vi "test_UDP Protocol Factory.vi"(8 "error in (no error)":errorcluster, 11 "TestCase in":refnum<class "Instrument Addon Scripting API Protocol Factories Unit Tests.lvclass">) -> (0 "error out":errorcluster, 3 "TestCase out":refnum<class "Instrument Addon Scripting API Protocol Factories Unit Tests.lvclass">)   [LabVIEW 2018, in "Instrument Addon Scripting API Protocol Factories Unit Tests.lvclass"]
uses:
  Instrument Addon Scripting API Protocol Factories Unit Tests.lvclass
  UDP/UDP Settings.ctl
  UDP/UDP.lvclass/UDP.ctl
  UDP/Data Access/Read Local IP Address.vi
  UDP/Data Access/Read Local Port.vi
  UDP/Data Access/Read Target IP Address.vi
  UDP/Data Access/Read Target Port.vi
  <vilib>/addons/_JKI Toolkits/VI Tester/TestCase.llb/TestCase.lvclass
  UDP/UDP.lvclass
  C:/Program Files (x86)/National Instruments/LabVIEW 2018/vi.lib/addons/_JKI Toolkits/VI Tester/TestCase.llb/TestCase.lvclass
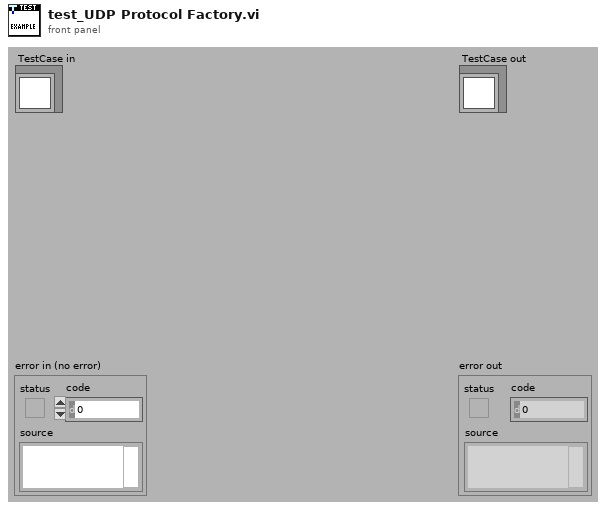
[diagram p1: front panel]
types:
  T1 = typedef "Protocols.lvlib/UDP.lvclass/UDP Settings.ctl" = cluster{"Local IP Address":string, "Local Port":u16, "Target IP Address":string, "Target Port":u16}
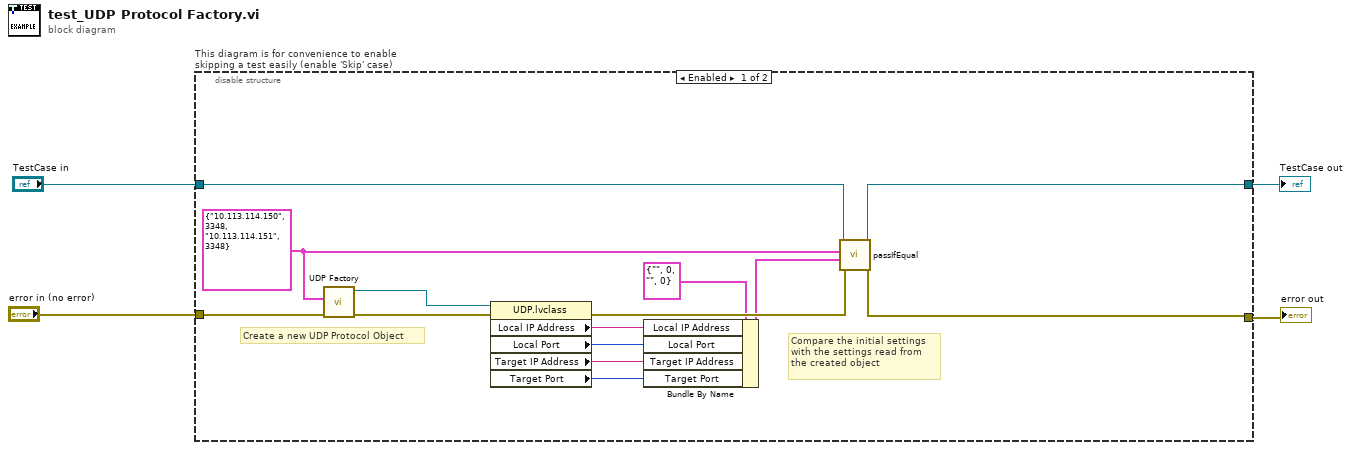
[diagram p0: block diagram]
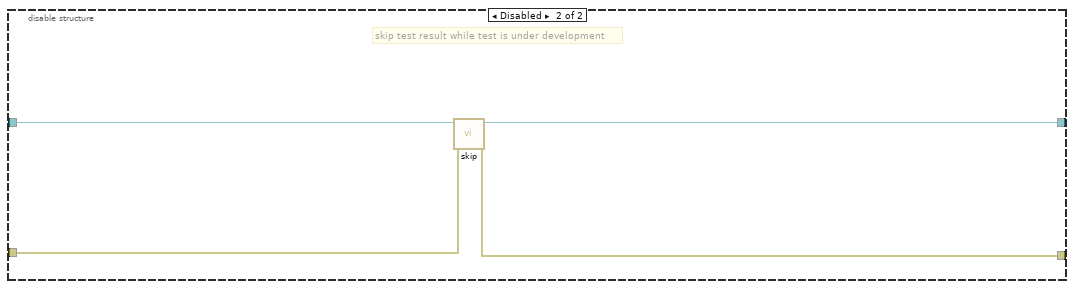
[diagram p2: hidden frame]
diagram:
  n1 = disable-structure "This diagram is for convenience to enable skipping a test easily (enable 'Skip' case)" shown="Enabled" {
    disable-tunnel: "TestCase in" -> [w18 w22]
    disable-tunnel: [w17 w20] -> w1
    disable-tunnel: [w16 w21] -> w3
    disable-tunnel: "error in (no error)" -> [w15 w19]
    frame Enabled {
      w13 = T1 {"Local IP Address"="10.113.114.150", "Local Port"=3348, "Target IP Address"="10.113.114.151", "Target Port"=3348} ("UPD Settings")
      # "Compare the initial settings \nwith the settings read from \nthe created object"
      # "Create a new UDP Protocol Object"
      n2 = call "UDP Factory.vi"("error in"=w15, "UPD Settings"=w13) -> ("error out"=w14:errorcluster, "UDP Out"=w12:refnum<class "UDP.lvclass">)  [unwired: 8 in]
      n3 = property class="UDP.lvclass"(reference=w12, error in=w14) -> (error out=w7:errorcluster, "Local IP Address"=w11:string, "Local Port"=w10:u16, "Target IP Address"=w9:string, "Target Port"=w8:u16)  [unwired: 1 out]
      n4 = Bundle By Name(cluster=T1 {"Local IP Address"="", "Local Port"=0, "Target IP Address"="", "Target Port"=0} ("UPD Settings"), "Local IP Address"=w11, "Local Port"=w10, "Target IP Address"=w9, "Target Port"=w8) -> (w5:T1)
      n5 = call-dynamic "passIfEqual.vi"("error in (no error)"=w7, "y"=w5, "x"=w13, "TestCase in"=w18) -> ("error out"=w16:errorcluster, "TestCase out"=w17:refnum<class "Instrument Addon Scripting API Protocol Factories Unit Tests.lvclass">)  [unwired: 6 in]
    }
    frame Disabled {
      # "skip test result while test is under development"
      n6 = call <vilib>:"skip.vi"("error in (no error)"=w19, "TestCase in"=w22) -> ("error out"=w21:errorcluster, "TestCase out"=w20:refnum<class "Instrument Addon Scripting API Protocol Factories Unit Tests.lvclass">)  [unwired: 8 in]
    }
  }
  "error out" <- w3
  "TestCase out" <- w1
